vi "Predefinied Event.vi"   [LabVIEW 2019, in "Events.lvclass"]
uses:
  Events.lvclass
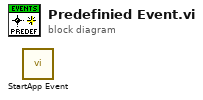
[diagram p0: block diagram]
diagram:
  n1 = call "StartApp Event.vi"() -> ()  [unwired: 10 in, 2 out]
